vi "fwd cheesy drive.vi"(4 "Loop Timer":i32=20, 6 "Time to stop":i32=300, 8 "Distance":dbl, 9 "Encoder Left":dbl, 10 "Encoder Right":dbl, 11 "Yaw":dbl) -> (0 "Finished distance":bool, 1 "Both finished":bool, 2 "Direction":dbl, 3 "Trottle":dbl)   [LabVIEW 2017]
panel:
  # "0,009\n0,025"
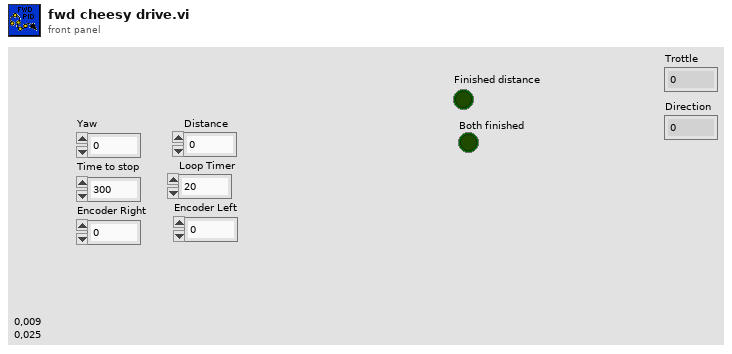
[diagram p1: front panel]
types:
  T1 = cluster{"proportional gain (Kc)":dbl, "integral time (Ti, min)":dbl, "derivative time (Td, min)":dbl}
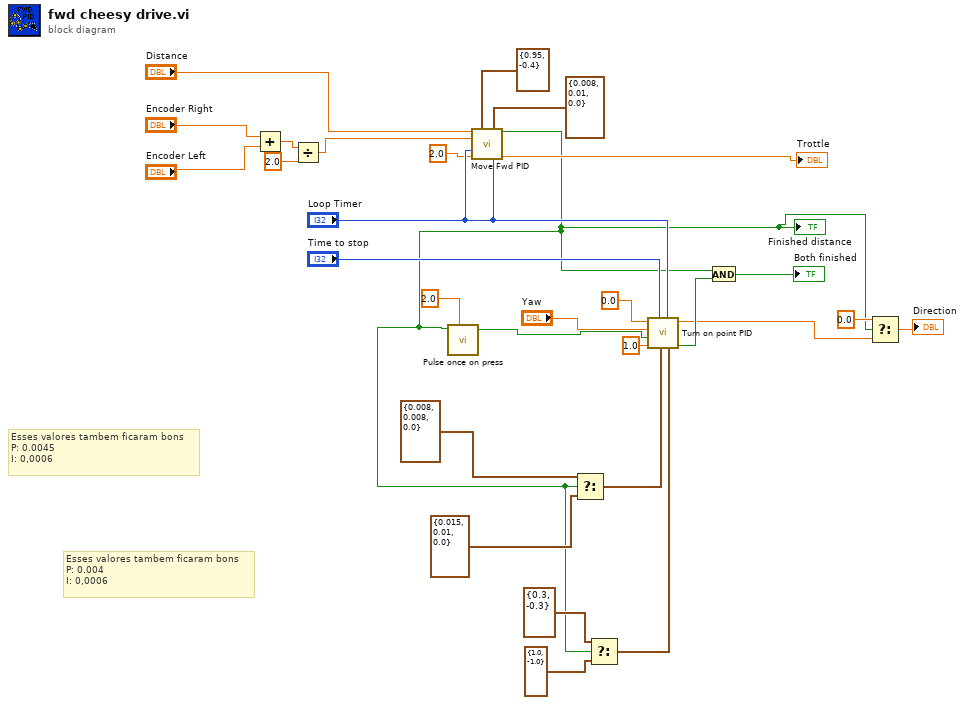
[diagram p0: block diagram]
diagram:
  # "Esses valores tambem ficaram bons\nP: 0.0045\nI: 0,0006"
  # "Esses valores tambem ficaram bons\nP: 0.004\nI: 0,0006"
  n1 = Add(x="Encoder Right", y="Encoder Left") -> (x+y=w21:dbl)
  n2 = Divide(x=w21, y=2.0) -> (x/y=w15:dbl)
  n3 = call "Move Fwd PID.vi"("Distance"="Distance", "Range"=cluster{"output high":dbl, "output low":dbl} {"output high"=0.95, "output low"=-0.4}, "Gains"=T1 {"proportional gain (Kc)"=0.008, "integral time (Ti, min)"=0.01, "derivative time (Td, min)"=0.0}, "Encoder Count"=w15, "Time to stop"="Loop Timer", "Precision"=2.0, "Loop Timer"="Loop Timer") -> ("Finished?"=w1:bool, "Output"=→"Trottle":dbl)  [unwired: 7 in]
  "Finished distance" <- w1
  n4 = call "Pulse once on press.vi"("in"=w1, "duration of pulse"=2.0) -> ("pulse"=w8:bool)  [unwired: 6 in]
  n5 = Select(t=T1 {"proportional gain (Kc)"=0.008, "integral time (Ti, min)"=0.008, "derivative time (Td, min)"=0.0} ("Gains"), s=w1, f=T1 {"proportional gain (Kc)"=0.015, "integral time (Ti, min)"=0.01, "derivative time (Td, min)"=0.0} ("Gains")) -> (s? t:f=w5:T1)
  n6 = Select(t=cluster{"output high":dbl, "output low":dbl} {"output high"=0.3, "output low"=-0.3} ("Range"), s=w1, f=cluster{"output high":dbl, "output low":dbl} {"output high"=1.0, "output low"=-1.0} ("Range")) -> (s? t:f=w3:cluster{"output high":dbl, "output low":dbl})
  n7 = call "Turn on point PID.vi"("Range"=w3, "Loop Timer"="Loop Timer", "Gains"=w5, "Time to stop"="Time to stop", "Precision"=1.0, "Reset"=w8, "Yaw"="Yaw", "Setpoint(degrees)"=0.0) -> ("Finished?"=w19:bool, "PWM left"=w10:dbl)  [unwired: 1 in, 1 out]
  n8 = And(x=w1, y=w19) -> (x .and. y?=→"Both finished":bool)
  n9 = Select(t=0.0, s=w1, f=w10) -> (s? t:f=→"Direction":dbl)
